vi "Stop Core.vi"(10 "final error code":i32, 11 "Air Cooler Application in":refnum<class "Air Cooler Application.lvclass">) -> (3 "Air Cooler Application out":refnum<class "Air Cooler Application.lvclass">)   [LabVIEW 2025, in "Air Cooler Application.lvlib" / "Air Cooler Application.lvclass"]
doc: "Perform any work needed when stopping the actor."
uses:
  Air Cooler Application.lvclass
  Air Cooler Application.lvclass/Air Cooler Application.ctl
  <vilib>/ActorFramework/Stop Msg/Stop Msg.lvclass/Stop Msg.ctl
  <vilib>/ActorFramework/Message Enqueuer/Message Enqueuer.lvclass/Message Enqueuer.ctl
  <vilib>/ActorFramework/Stop Msg/Send Emergency Stop.vi
  <vilib>/ActorFramework/Stop Msg/Send Normal Stop.vi
  <vilib>/ActorFramework/Message Enqueuer/Enqueue Critical.vi
  <vilib>/ActorFramework/Message Enqueuer/Enqueue.vi
  <vilib>/ActorFramework/Stop Msg/Stop Msg.lvclass
  C:/Program Files/National Instruments/LabVIEW 2025/vi.lib/ActorFramework/Message/Message.lvclass
  <vilib>/ActorFramework/Message Priority Queue/Priority Enqueue.vi
  <vilib>/ActorFramework/Actor/Actor.lvclass
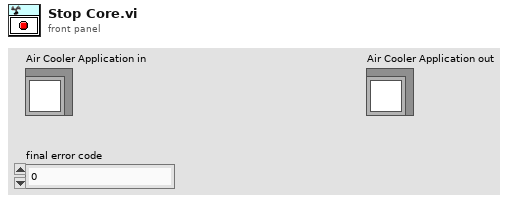
[diagram p1: front panel]
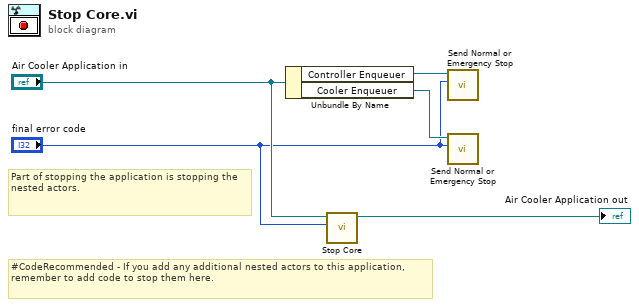
[diagram p0: block diagram]
diagram:
  # "#CodeRecommended - If you add any additional nested actors to this application, remember to add code to stop them here."
  # "Part of stopping the application is stopping the nested actors."
  n1 = Unbundle By Name("Air Cooler Application in") -> ("Controller Enqueuer"=w3:refnum<class "Message Enqueuer.lvclass">, "Cooler Enqueuer"=w2:refnum<class "Message Enqueuer.lvclass">)
  n2 = call-parent "Stop Core.vi"("final error code"="final error code", "Actor in"="Air Cooler Application in") -> ("Actor out"=→"Air Cooler Application out":refnum<class "Air Cooler Application.lvclass">)  [unwired: 9 in]
  n3 = call <vilib>:"Send Normal or Emergency Stop.vi"("final error code"="final error code", "Message Enqueuer"=w3) -> ()  [unwired: 9 in, 1 out]
  n4 = call <vilib>:"Send Normal or Emergency Stop.vi"("final error code"="final error code", "Message Enqueuer"=w2) -> ()  [unwired: 9 in, 1 out]
